vi "LUCS001RT_GPS_Decoder_GPGGA.vi"(8 "error in (no error)":errorcluster, 9 "SerialData: GPGLL":string=",170834,4124.8963,N,08151.6838,W,1,05,1.5,280.2,M,-34.0,M,,,*75 \n", 11 "GPS Data In":T1={"WayPointDataGood"=TRUE, "Waypoint:XTE"=0.01, "Waypoint:SteeringDirection"="L", "WayPoint:OriginID"="", "Waypoint:DestinationID"="", "DestinationWaypoint.Latitude.Deg"=0, "DestinationWaypoint.Latitude.Min"=0.0, "DestinationWaypointLatitude.North/South"="", "DestinationWaypointLongitude.Deg"=0, "DestinationWaypointLongitude.Min"=0.0, "DestinationWaypointLongitude.East/West"="", "RangeToDestination(NauticalMiles)"=0.0, "TrueBearingToDestination"=33.7, "VelocityTowardsDestination(Knots)"=0.0, "ArrivalAlarm"=TRUE, "ITOW"=247, "TAcc"=0, "LON"=0.0, "LAT"=0.0, "HEIGHT"=0, "HMSL"=0, "Hacc"=0, "Vacc"=0, "MSTOW"=0, "FixType"=0, "ECEF_X_Coor"=0, "ECEF_Y_Coor"=0, "ECEF_Z_Coor"=0, "Pacc"=0, "ECEF_X_Vlsty"=0, "ECEF_Y_Vlsty"=0, "ECEF_Z_Vlsty"=0, "Sacc"=0, "PosDOP"=0, "#SatsInNavSol"=0, "NED_NVsty"=0, "NED_Evsty"=0, "NED_DNvsty"=0, "Speed(3-D)"=0, "GSpeed(2-D)"=0, "Heading(2-D)"=0.0, "CAcc"=0, "Nano"=0, "Year"=0, "Month"=0, "Day"=0, "Hour"=0, "Min"=0, "Sec"=0, "UTC Valid"=0} {"UTC Valid" items=["UTC not valid", "Valid Time of Week", "Valid Week Number", "NA", "Valid UTC"]; "CAcc" format="%.0f°"; "Heading(2-D)" format="%0.6f°"; "GSpeed(2-D)" format="%.0f cm/s"; "Speed(3-D)" format="%.0f cm/s"; "NED_DNvsty" format="%.0f cm/s"; "NED_Evsty" format="%.0f cm/s"; "NED_NVsty" format="%.0f cm/s"; "Sacc" format="%.0f cm/s"; "ECEF_Z_Vlsty" format="%.0f cm/s"; "ECEF_Y_Vlsty" format="%.0f cm/s"; "ECEF_X_Vlsty" format="%.0f cm/s"; "FixType" items=["No Fix", "Dead Reckoning Only", "2D-Fix", "3D-Fix", "GPS + Dead Reckoning", "Time Only Fix", "RESERVED"]; "Vacc" format="%.0f mm"; "Hacc" format="%.0f mm"; "HMSL" format="%d mm"; "HEIGHT" format="%.0f mm"; "LAT" format="%#.6f"; "LON" format="%#.6f"; "Waypoint:XTE" format="%#.2f"}) -> (0 "error out":errorcluster, 3 "GPS Data Out":T1={"WayPointDataGood"=TRUE, "Waypoint:XTE"=0.01, "Waypoint:SteeringDirection"="L", "WayPoint:OriginID"="", "Waypoint:DestinationID"="", "DestinationWaypoint.Latitude.Deg"=0, "DestinationWaypoint.Latitude.Min"=0.0, "DestinationWaypointLatitude.North/South"="", "DestinationWaypointLongitude.Deg"=0, "DestinationWaypointLongitude.Min"=0.0, "DestinationWaypointLongitude.East/West"="", "RangeToDestination(NauticalMiles)"=0.0, "TrueBearingToDestination"=33.7, "VelocityTowardsDestination(Knots)"=0.0, "ArrivalAlarm"=TRUE, "ITOW"=247, "TAcc"=0, "LON"=0.0, "LAT"=16.0, "HEIGHT"=0, "HMSL"=0, "Hacc"=0, "Vacc"=0, "MSTOW"=0, "FixType"=0, "ECEF_X_Coor"=0, "ECEF_Y_Coor"=0, "ECEF_Z_Coor"=0, "Pacc"=0, "ECEF_X_Vlsty"=0, "ECEF_Y_Vlsty"=0, "ECEF_Z_Vlsty"=0, "Sacc"=0, "PosDOP"=0, "#SatsInNavSol"=0, "NED_NVsty"=0, "NED_Evsty"=0, "NED_DNvsty"=0, "Speed(3-D)"=0, "GSpeed(2-D)"=0, "Heading(2-D)"=0.0, "CAcc"=0, "Nano"=0, "Year"=0, "Month"=0, "Day"=0, "Hour"=0, "Min"=0, "Sec"=0, "UTC Valid"=0} {"UTC Valid" items=["UTC not valid", "Valid Time of Week", "Valid Week Number", "NA", "Valid UTC"]; "CAcc" format="%.0f°"; "Heading(2-D)" format="%0.6f°"; "GSpeed(2-D)" format="%.0f cm/s"; "Speed(3-D)" format="%.0f cm/s"; "NED_DNvsty" format="%.0f cm/s"; "NED_Evsty" format="%.0f cm/s"; "NED_NVsty" format="%.0f cm/s"; "Sacc" format="%.0f cm/s"; "ECEF_Z_Vlsty" format="%.0f cm/s"; "ECEF_Y_Vlsty" format="%.0f cm/s"; "ECEF_X_Vlsty" format="%.0f cm/s"; "FixType" items=["No Fix", "Dead Reckoning Only", "2D-Fix", "3D-Fix", "GPS + Dead Reckoning", "Time Only Fix", "RESERVED"]; "Vacc" format="%.0f mm"; "Hacc" format="%.0f mm"; "HMSL" format="%d mm"; "HEIGHT" format="%.0f mm"; "LAT" format="%#.6f"; "LON" format="%#.6f"; "Waypoint:XTE" format="%#.2f"})   [LabVIEW 2024]
uses:
  LUCS001RT_GPS_Data.ctl
panel:
  # "WAYPOINT"
  # "CURRENT POSITION"
  # "WAYPOINT"
  # "CURRENT POSITION"
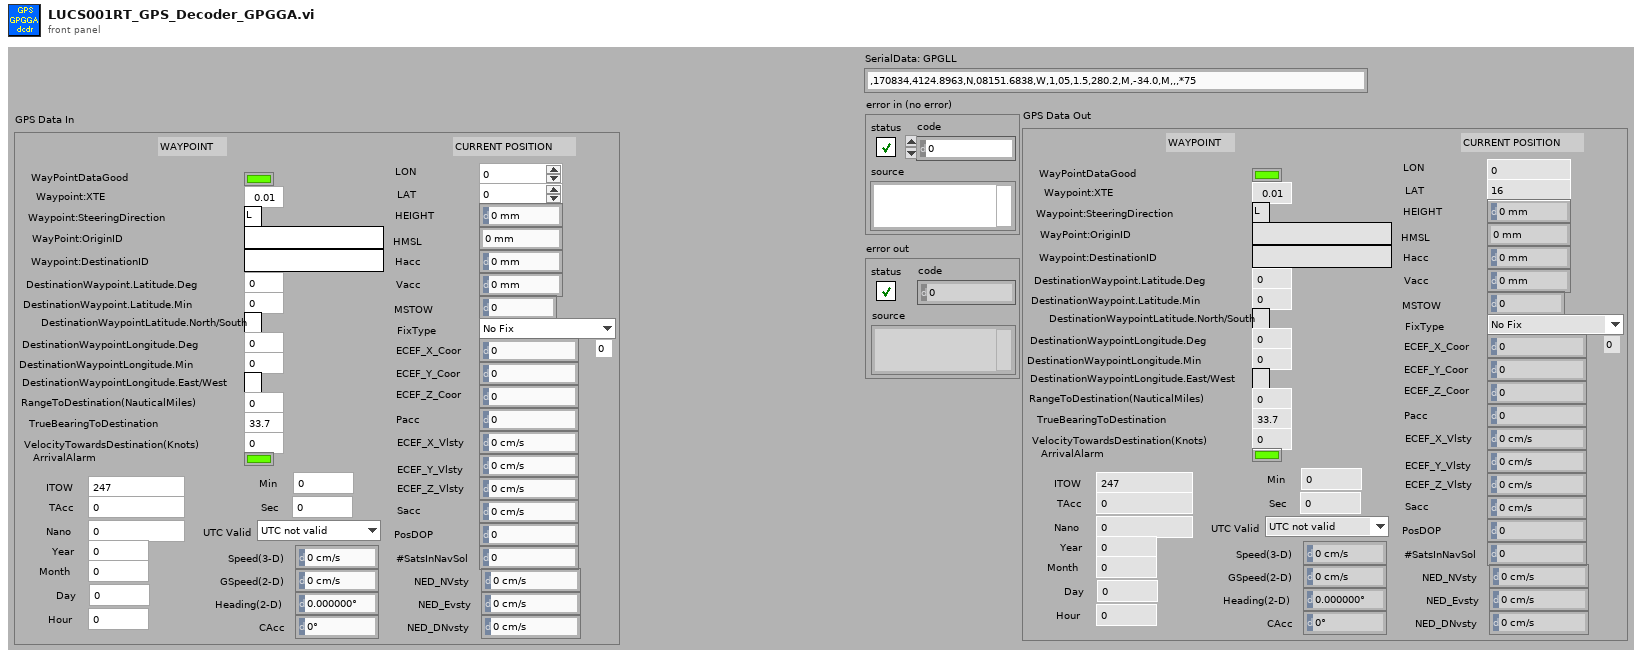
[diagram p1: front panel]
types:
  T1 = typedef "LUCS001RT_GPS_Data.ctl" = cluster{"WayPointDataGood":bool, "Waypoint:XTE":dbl, "Waypoint:SteeringDirection":string, "WayPoint:OriginID":string, "Waypoint:DestinationID":string, "DestinationWaypoint.Latitude.Deg":i32, "DestinationWaypoint.Latitude.Min":dbl, "DestinationWaypointLatitude.North/South":string, "DestinationWaypointLongitude.Deg":i32, "DestinationWaypointLongitude.Min":dbl, "DestinationWaypointLongitude.East/West":string, "RangeToDestination(NauticalMiles)":dbl, "TrueBearingToDestination":dbl, "VelocityTowardsDestination(Knots)":dbl, "ArrivalAlarm":bool, "ITOW":u32, "TAcc":u32, "LON":dbl, "LAT":dbl, "HEIGHT":i32, "HMSL":i32, "Hacc":u32, "Vacc":u32, "MSTOW":u32, "FixType":u8, "ECEF_X_Coor":i32, "ECEF_Y_Coor":i32, "ECEF_Z_Coor":i32, "Pacc":u32, "ECEF_X_Vlsty":i32, "ECEF_Y_Vlsty":i32, "ECEF_Z_Vlsty":i32, "Sacc":u32, "PosDOP":u16, "#SatsInNavSol":u8, "NED_NVsty":i32, "NED_Evsty":i32, "NED_DNvsty":i32, "Speed(3-D)":u32, "GSpeed(2-D)":u32, "Heading(2-D)":dbl, "CAcc":u32, "Nano":i32, "Year":u16, "Month":u8, "Day":u8, "Hour":u8, "Min":u8, "Sec":u8, "UTC Valid":u8}
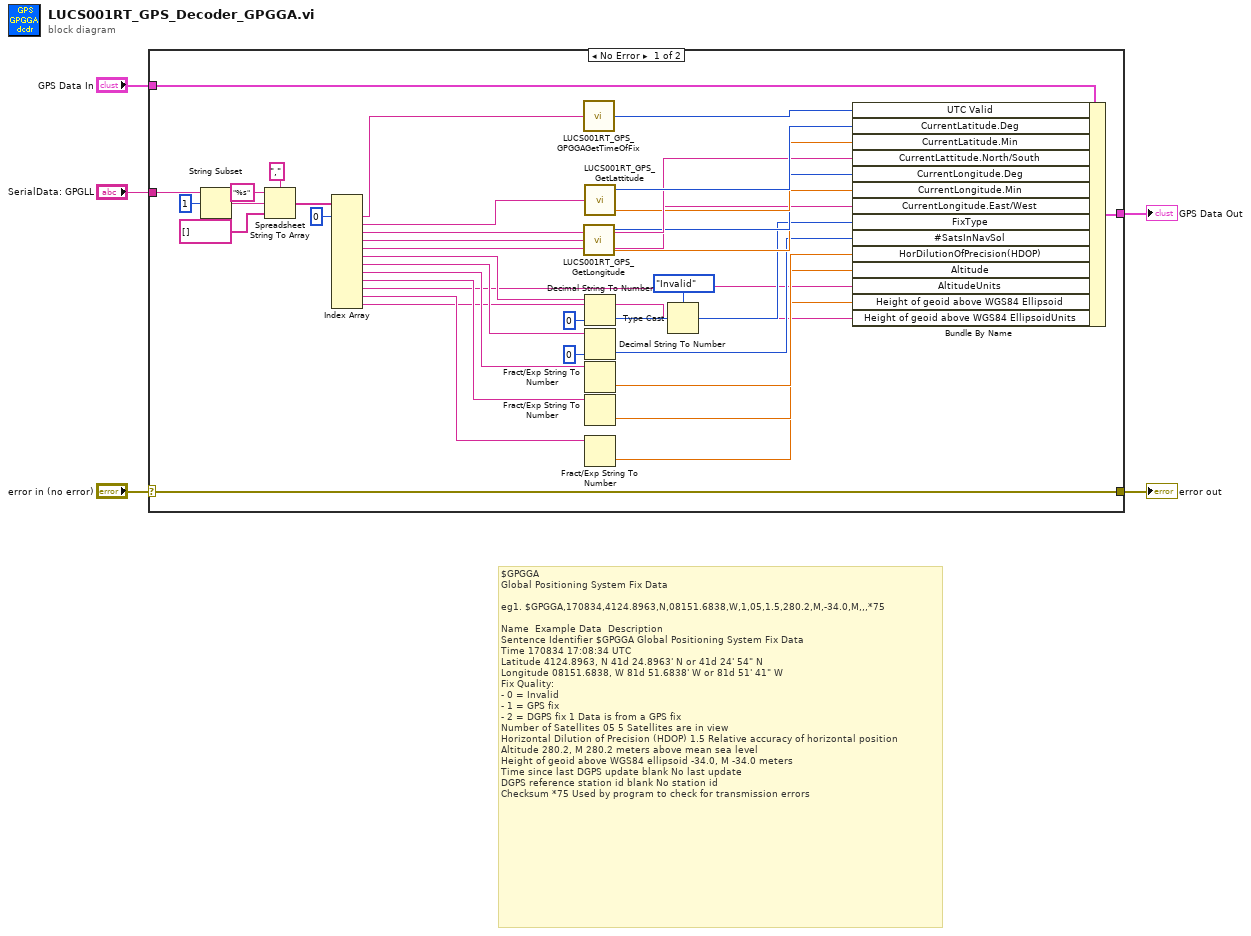
[diagram p0: block diagram]
diagram:
  # "$GPGGA\nGlobal Positioning System Fix Data \n\neg1. $GPGGA,170834,4124.8963,N,08151.6838,W,1,05,1.5,280.2,M,-34.0,M,,,*75 \n\nName  Example Data  Description  \nSentence Identifier $GPGGA Global Positioning System Fix Data \nTime 170834 17:08:34 UTC \nLatitude 4124.8963, N 41d 24.8963' N or 41d 24' 54\" N \nLongitude 08151.6838, W 81d 51.6838' W or 81d 51' 41\" W \nFix Quality:\n- 0 = Invalid\n- 1 = GPS fix\n- 2 = DGPS fix 1 Data is from a GPS fix \nNumber of Satellites 05 5 Satellites are in view \nHorizontal Dilution of Precision (HDOP) 1.5 Relative accuracy of horizontal position \nAltitude 280.2, M 280.2 meters above mean sea level \nHeight of geoid above WGS84 ellipsoid -34.0, M -34.0 meters \nTime since last DGPS update blank No last update \nDGPS reference station id blank No station id \nChecksum *75 Used by program to check for transmission errors"
  n1 = case shown="No Error" "error in (no error)" {
    selector: "error in (no error)" -> [w33 w43]
    tunnel: "SerialData: GPGLL" -> [w7 _]
    tunnel: "GPS Data In" -> [w9 _]
    tunnel: [w35 _] -> w3
    tunnel: [w33 w43] -> w1
    frame No Error {
      n2 = String Subset(string=w7, offset (0)=1) -> (substring=w38:string)  [unwired: 1 in]
      n3 = Spreadsheet String To Array(delimiter (Tab)=",", format string="%s", spreadsheet string=w38, array type (2D Dbl)=string[] []) -> (array=w42:string[])
      n4 = Index Array(array=w42, index #1=0 ("index")) -> (element #1=w8:string, element #2=w28:string, element #3=w32:string, element #4=w27:string, element #5=w26:string, element #6=w25:string, element #7=w19:string, element #8=w17:string, element #9=w15:string, element #10=w13:string, element #11=w12:string, element #12=w10:string)  [unwired: 11 in]
      n5 = call "LUCS001RT_GPS_GPGGAGetTimeOfFix.vi"("String:CurrentPosition.TimeOfFix"=w8) -> ("CurrentPosition.TimeOfFix"=w6:u32)  [unwired: 6 in]
      n6 = call "LUCS001RT_GPS_GetLongitude.vi"("LongitudeString"=w27) -> ("Longitude.Degrees"=w30:i32, "Longitude.Minutes"=w29:dbl)  [unwired: 5 in]
      n7 = call "LUCS001RT_GPS_GetLattitude.vi"("LattitudeString"=w28) -> ("Lattitude.Degrees"=w34:i32, "Lattitude.Minutes"=w31:dbl)  [unwired: 5 in]
      n8 = Decimal String To Number(string=w25, default (0L)=u8 0 ("default (0 I32)")) -> (number=w22:u8)  [unwired: 1 in, 1 out]
      n9 = Decimal String To Number(string=w19, default (0L)=u8 0 ("default (0 I32)")) -> (number=w18:u8)  [unwired: 1 in, 1 out]
      n10 = Fract/Exp String To Number(string=w17) -> (number=w16:dbl)  [unwired: 3 in, 1 out]
      n11 = Fract/Exp String To Number(string=w15) -> (number=w14:dbl)  [unwired: 3 in, 1 out]
      n12 = Fract/Exp String To Number(string=w12) -> (number=w11:dbl)  [unwired: 3 in, 1 out]
      n13 = Type Cast(type=enum8{"Invalid", "GPS Fix", "DGPS Fix 1"}."Invalid" ("FixQuality"), x=w22) -> (*(type *) &x=w21:enum8{"Invalid", "GPS Fix", "DGPS Fix 1"})
      n14 = Bundle By Name(cluster=w9, "UTC Valid"=w6, "CurrentLatitude.Deg"=w34, "CurrentLatitude.Min"=w31, "CurrentLattitude.North/South"=w32, "CurrentLongitude.Deg"=w30, "CurrentLongitude.Min"=w29, "CurrentLongitude.East/West"=w26, "FixType"=w21, "#SatsInNavSol"=w18, "HorDilutionOfPrecision(HDOP)"=w16, "Altitude"=w14, "AltitudeUnits"=w13, "Height of geoid above WGS84 Ellipsoid"=w11, "Height of geoid above WGS84 EllipsoidUnits"=w10) -> (w35:T1)
    }
    frame Error {
    }
  }
  "GPS Data Out" <- w3
  "error out" <- w1
